vi "BMU参数读取-Auto.vi"(7 "Socket":dbl, 8 "CAN端口":u16(ring), 9 "设备索引号":u16(ring), 10 "CAN卡类型":u32(ring)=21, 11 "从板号":u8=1) -> (3 "成功?":bool)   [LabVIEW 2013] (continued)
                                n1965 = control-ref of="二维码信息"() -> (w3309:refnum<vi>)
                                n1966 = local write "主板数据"(w3310) -> ()
                                }
                                frame #1 {
                                n1967 = control-ref of="主板数据"() -> (w3321:refnum<vi>)
                                }
                                }
                                }
                                frame "从板" {
                                n1968 = stacked-sequence {
                                tunnel: [_ w3333] -> w3322
                                frame #0 {
                                n1969 = control-ref of="从板号"() -> (w3327:refnum<vi>)
                                n1970 = control-ref of="项目信息 2"() -> (w3328:refnum<vi>)
                                n1971 = control-ref of="电池组信息"() -> (w3326:refnum<vi>)
                                n1972 = control-ref of="加热控制参数"() -> (w3329:refnum<vi>)
                                n1973 = control-ref of="一级故障(从板)"() -> (w3330:refnum<vi>)
                                n1974 = control-ref of="二级故障(从板)"() -> (w3331:refnum<vi>)
                                n1975 = control-ref of="三级故障(从板)"() -> (w3332:refnum<vi>)
                                n1976 = control-ref of="均衡参数"() -> (w3325:refnum<vi>)
                                n1977 = local read "从板信息"() -> (w3324:T2)
                                n1978 = Bundle(cluster=w3324, "从板号"=w3327, "项目信息 2"=w3328, "加热控制参数"=w3329, "一级故障(从板)"=w3330, "二级故障(从板)"=w3331, "三级故障(从板)"=w3332, "电池组信息(从板)"=w3326, "均衡参数"=w3325) -> (w3323:T2)
                                n1979 = local write "从板信息"(w3323) -> ()
                                }
                                frame #1 {
                                n1980 = control-ref of="从板信息"() -> (w3333:refnum<vi>)
                                }
                                }
                                }
                              }
                              n1981 = control-ref of="BMU读取结果"() -> (w3294:refnum<vi>)
                              n1982 = control-ref of="二维码信息 2"() -> (w3296:refnum<vi>)
                              n1983 = control-ref of="结果"() -> (w3303:refnum<vi>)
                              n1984 = control-ref of="从板个数"() -> (w3299:refnum<vi>)
                              n1985 = call "输出数据解析.vi"("主板引用"=w3301, "错误代码"=w3306, "BMU读取结果"=w3294, "命令序号"=w3305, "输入数组"=w3304, "命令"=w3302, "从板引用"=w3300, "进度引用"=w3303, "板选择"=w3298, "从板个数"=w3299, "二维码信息"=w3297, "从板二维码信息"=w3296) -> ("写入超时"=→"写入超时":bool)  [unwired: 4 in, 3 out]
                            }
                            frame True {
                              n1986 = Index Array(array=w3334, index #1=0 ("索引"), index #2=1 ("索引")) -> (element #1=w3337:u8, element #2=w3338:u8)
                              n1987 = Join Numbers(hi=w3337, lo=w3338) -> ((hi.lo)=w3336:u16)
                              n1988 = Number To Hexadecimal String(2:w3336) -> (0:w3335:string)  [unwired: 1 out]
                              n1989 = control-ref of="结果"() -> (w3343:refnum<vi>)
                              n1990 = Concatenate Strings("0x" ("字符串"), w3335) -> (w3344:string)
                              n1991 = Build Array(w3344) -> (w3345:string[])
                              n1992 = call "表格编辑.vi"("新元素/子数组"=w3345, "活动单元格:单元格背景色"=u32 16740749, "MCListbox引用句柄"=w3343) -> ()  [unwired: 9 out]
                            }
                          }
                          n1993 = global write "EV05全局变量1.vi" "流控帧 2"(FALSE ("流控帧 2")) -> ()
                          n1994 = global write "EV05全局变量1.vi" "输出数组"(i32[] []) -> ()
                          n1995 = local write "控制1"(FALSE ("控制1")) -> ()
                          n1996 = local write "消除"(FALSE ("消除")) -> ()
                        }
                      }
                    }
                    frame True {
                      # "写参数判定"
                      n1997 = And(x="控制1", y=w3351) -> (x .and. y?=w3348:bool)
                      n1998 = case shown="真" w3348 {
                        tunnel: w3350 -> [_ w3358]
                        tunnel: w3349 -> [_ w3355]
                        frame False {
                        }
                        frame True {
                          n1999 = call <vilib>:"Unset Busy.vi"() -> ()  [unwired: 2 in, 10 out]
                          n2000 = case shown="\"主板\", 默认" w3355 {
                            tunnel: [w3359 w3360] -> w3357
                            frame "主板", Default {
                              n2001 = local read "主板选项"() -> (w3359:string)
                            }
                            frame "从板" {
                              n2002 = local read "从板选项"() -> (w3360:string)
                            }
                          }
                          n2003 = control-ref of="结果"() -> (w3356:refnum<vi>)
                          n2004 = call "输入数据判定.vi"("主从选择"=w3355, "主板选项"=w3357, "进度引用"=w3356, "错误代码"=w3358) -> ()  [unwired: 3 in, 5 out]
                          n2005 = global write "EV05全局变量1.vi" "流控帧 2"(FALSE ("流控帧 2")) -> ()
                          n2006 = local write "控制1"(FALSE ("控制1")) -> ()
                          n2007 = local write "消除"(FALSE ("消除")) -> ()
                        }
                      }
                      n2008 = global write "EV05全局变量1.vi" "输出数组"(i32[] []) -> ()
                    }
                  }
                }
                frame "版本读取" {
                  n2009 = local read "命令序号"() -> (w3361:u8)
                  n2010 = local read "从板板号"() -> (w3364:u8)
                  n2011 = local read "控制1"() -> (w3365:bool)
                  n2012 = call "多帧接收机制(EV05).vi"("can卡类型"=w3372, "设备索引号"=w3371, "CAN端口"=w3370, "VCI_Receive"=w3369, "命令"=w3368, "板号"=w3364, "命令序号"=w3361) -> ("错误信号"=w3362:bool, "输出数组"=w3373:u8[], "读错误代码"=w3363:u8[], "结束信号"=w3367:bool)  [unwired: 3 in, 6 out]
                  n2013 = And(x=w3365, y=w3367) -> (x .and. y?=w3366:bool)
                  n2014 = case shown="真" w3366 {
                    tunnel: w3373 -> [_ w3381]
                    tunnel: w3361 -> [_ w3380]
                    tunnel: w3368 -> [_ w3379]
                    tunnel: w3363 -> [_ w3375]
                    tunnel: w3362 -> [_ w3374]
                    frame False {
                    }
                    frame True {
                      n2015 = case shown="假" w3374 {
                        tunnel: w3381 -> [w3385 _]
                        tunnel: w3380 -> [w3384 _]
                        tunnel: w3379 -> [w3383 _]
                        tunnel: w3375 -> [w3382 w3609]
                        frame False {
                          n2016 = case shown="89" w3383 {
                            tunnel: w3384 -> [_ w3388]
                            tunnel: w3385 -> [_ w3387]
                            tunnel: w3382 -> [_ _]
                            frame 0, Default {
                            }
                            frame 137 {
                              n2017 = case shown="1" w3388 {
                                tunnel: w3387 -> [_ w3416 w3460 w3480 w3607]
                                frame 0, Default {
                                }
                                frame 1 {
                                w3398 = "." ("字符串")
                                n2018 = Array Subset(array=w3416, index=0 ("索引"), length=14 ("长度")) -> (w3429:u8[])
                                n2019 = Index Array(array=w3416, index=14 ("索引")) -> (element=w3419:u8)
                                n2020 = Index Array(array=w3416, index #1=15 ("索引"), index #2=16 ("索引")) -> (element #1=w3425:u8, element #2=w3426:u8)
                                n2021 = Index Array(array=w3416, index #1=17 ("索引"), index #2=18 ("索引")) -> (element #1=w3420:u8, element #2=w3421:u8)
                                n2022 = call "数组去零.vi"("输入"=w3429) -> ("输出"=w3404:dbl[])
                                n2023 = Join Numbers(hi=w3420, lo=w3421) -> ((hi.lo)=w3417:u16)
                                n2024 = Join Numbers(hi=w3425, lo=w3426) -> ((hi.lo)=w3418:u16)
                                n2025 = Number To Decimal String(number=w3419) -> (decimal integer string=w3411:string)  [unwired: 1 out]
                                n2026 = Byte Array To String(unsigned byte array=w3404) -> (string=w3403:string)
                                n2027 = Number To Decimal String(number=w3417) -> (decimal integer string=w3399:string)  [unwired: 1 out]
                                n2028 = Number To Decimal String(number=w3418) -> (decimal integer string=w3410:string)  [unwired: 1 out]
                                n2029 = Array Subset(array=w3416, index=21 ("索引"), length=7 ("长度")) -> (w3413:u8[])
                                n2030 = Concatenate Strings("V" ("字符串"), w3411, w3398, w3410, w3398, w3399) -> (w3408:string)
                                n2031 = call "数组去零.vi"("输入"=w3413) -> ("输出"=w3396:dbl[])
                                n2032 = Byte Array To String(unsigned byte array=w3396) -> (string=w3394:string)
                                n2033 = call <vilib>:"Space Constant.vi"() -> ("String"=w3395:string)
                                n2034 = Equal?(x=w3394, y=w3395) -> (x = y?=w3400:bool)
                                n2035 = Concatenate Strings("-" ("字符串"), w3394) -> (w3401:string)
                                n2036 = Select(t=w3395, s=w3400, f=w3401) -> (s? t:f=w3397:string)
                                n2037 = Concatenate Strings(w3403, "-" ("字符串"), w3408, w3397) -> (w3390:string)
                                n2038 = local read "项目软件版本"() -> (w3392:string[])
                                n2039 = local read "从板板号"() -> (w3389:u8)
                                n2040 = local write "项目软件版本号"(w3390) -> ()
                                n2041 = Replace Array Subset(array=w3392, new element=w3390, index=w3389) -> (w3391:string[])
                                n2042 = control-ref of="结果"() -> (w3407:refnum<vi>)
                                n2043 = local write "项目软件版本"(w3391) -> ()
                                n2044 = Build Array("项目软件版本     读取完成" ("读取结果")) -> (w3405:string[])
                                n2045 = call "表格编辑(版本读取).vi"("新元素/子数组"=w3405, "活动单元格:单元格背景色"=u32 6618880, "MCListbox引用句柄"=w3407) -> ()  [unwired: 9 out]
                                }
                                frame 2 {
                                w3443 = ""
                                w3440 = "." ("字符串")
                                n2046 = Array Subset(array=w3460, index=0 ("索引"), length=14 ("长度")) -> (w3448:u8[])
                                n2047 = Index Array(array=w3460, index=14 ("索引")) -> (element=w3463:u8)
                                n2048 = Index Array(array=w3460, index #1=15 ("索引"), index #2=16 ("索引")) -> (element #1=w3469:u8, element #2=w3470:u8)
                                n2049 = Index Array(array=w3460, index #1=17 ("索引"), index #2=18 ("索引")) -> (element #1=w3464:u8, element #2=w3465:u8)
                                n2050 = Join Numbers(hi=w3464, lo=w3465) -> ((hi.lo)=w3461:u16)
                                n2051 = Join Numbers(hi=w3469, lo=w3470) -> ((hi.lo)=w3462:u16)
                                n2052 = Number To Decimal String(number=w3461) -> (decimal integer string=w3441:string)  [unwired: 1 out]
                                n2053 = call "数组去零.vi"("输入"=w3448) -> ("输出"=w3447:dbl[])
                                n2054 = Number To Decimal String(number=w3463) -> (decimal integer string=w3455:string)  [unwired: 1 out]
                                n2055 = Number To Decimal String(number=w3462) -> (decimal integer string=w3454:string)  [unwired: 1 out]
                                n2056 = Array Subset(array=w3460, index=21 ("索引"), length=7 ("长度")) -> (w3457:u8[])
                                n2057 = Byte Array To String(unsigned byte array=w3447) -> (string=w3442:string)
                                n2058 = call "数组去零.vi"("输入"=w3457) -> ("输出"=w3439:dbl[])
                                n2059 = Concatenate Strings("V" ("字符串"), w3455, w3440, w3454, w3440, w3441) -> (w3452:string)
                                n2060 = Byte Array To String(unsigned byte array=w3439) -> (string=w3437:string)
                                n2061 = Equal?(x=w3443, y=w3437) -> (x = y?=w3444:bool)
                                n2062 = Concatenate Strings("-" ("字符串"), w3437) -> (w3445:string)
                                n2063 = Select(t=w3443, s=w3444, f=w3445) -> (s? t:f=w3438:string)
                                n2064 = Concatenate Strings(w3442, "-" ("字符串"), w3452, w3438) -> (w3433:string)
                                n2065 = local read "平台软件版本"() -> (w3435:string[])
                                n2066 = local read "从板板号"() -> (w3432:u8)
                                n2067 = local write "平台软件版本号"(w3433) -> ()
                                n2068 = Replace Array Subset(array=w3435, new element=w3433, index=w3432) -> (w3434:string[])
                                n2069 = control-ref of="结果"() -> (w3450:refnum<vi>)
                                n2070 = local write "平台软件版本"(w3434) -> ()
                                n2071 = Build Array("平台软件版本     读取完成" ("读取结果")) -> (w3449:string[])
                                n2072 = call "表格编辑(版本读取).vi"("新元素/子数组"=w3449, "活动单元格:单元格背景色"=u32 6618880, "MCListbox引用句柄"=w3450) -> ()  [unwired: 1 in, 8 out]
                                }
                                frame 3 {
                                n2073 = Index Array(array=w3480, index #1=0 ("索引"), index #2=1 ("索引")) -> (element #1=w3476:u8, element #2=w3477:u8)
                                n2074 = Join Numbers(hi=w3476, lo=w3477) -> ((hi.lo)=w3475:u16)
                                n2075 = case shown="99, 默认" w3475 {
                                tunnel: w3480 -> [w3483 _ w3517]
                                tunnel: w3475 -> [_ _ w3495]
                                frame 0 {
                                n2076 = Index Array(array=w3483, index #1=2 ("索引"), index #2=3 ("索引")) -> (element #1=w3487:u8, element #2=w3486:u8)
                                n2077 = Join Numbers(hi=w3487, lo=w3486) -> ((hi.lo)=w3482:u16)
                                n2078 = for {
                                N: w3482 -> [_]
                                tunnel: w3483 -> [w3492]
                                tunnel: [w3488] -> w3481 mode=indexing
                                i -> [w3491]
                                n2079 = Add(x=w3491, y=4) -> (x+y=w3489:i32)
                                n2080 = Index Array(array=w3492, index=w3489) -> (element=w3488:u8)
                                }
                                "MODEL号" <- w3481
                                }
                                frame 99, Default {
                                }
                                frame 1..40 {
                                w3500 = ""
                                w3521 = "." ("字符串")
                                n2081 = Array Subset(array=w3517, index=2 ("索引"), length=14 ("长度")) -> (w3506:u8[])
                                n2082 = Index Array(array=w3517, index=16 ("索引")) -> (element=w3529:u8)
                                n2083 = Index Array(array=w3517, index #1=17 ("索引"), index #2=18 ("索引")) -> (element #1=w3535:u8, element #2=w3536:u8)
                                n2084 = Index Array(array=w3517, index #1=19 ("索引"), index #2=20 ("索引")) -> (element #1=w3530:u8, element #2=w3531:u8)
                                n2085 = Join Numbers(hi=w3530, lo=w3531) -> ((hi.lo)=w3527:u16)
                                n2086 = Join Numbers(hi=w3535, lo=w3536) -> ((hi.lo)=w3528:u16)
                                n2087 = Number To Decimal String(number=w3495) -> (decimal integer string=w3515:string)  [unwired: 1 out]
                                n2088 = Number To Decimal String(number=w3529) -> (decimal integer string=w3523:string)  [unwired: 1 out]
                                n2089 = call "数组去零.vi"("输入"=w3506) -> ("输出"=w3505:dbl[])
                                n2090 = Number To Decimal String(number=w3528) -> (decimal integer string=w3522:string)  [unwired: 1 out]
                                n2091 = Number To Decimal String(number=w3527) -> (decimal integer string=w3520:string)  [unwired: 1 out]
                                n2092 = Byte Array To String(unsigned byte array=w3505) -> (string=w3507:string)
                                n2093 = Concatenate Strings("第" ("读取结果"), w3515, "模块" ("字符串"), "     读取完成" ("读取结果")) -> (w3508:string)
                                n2094 = Concatenate Strings("V" ("字符串"), w3523, w3521, w3522, w3521, w3520) -> (w3518:string)
                                n2095 = control-ref of="结果"() -> (w3511:refnum<vi>)
                                n2096 = Array Subset(array=w3517, index=23 ("索引"), length=7 ("长度")) -> (w3504:u8[])
                                n2097 = call "数组去零.vi"("输入"=w3504) -> ("输出"=w3499:dbl[])
                                n2098 = Byte Array To String(unsigned byte array=w3499) -> (string=w3496:string)
                                n2099 = Build Array(w3508) -> (w3510:string[])
                                n2100 = control-ref of="模块软件版本 2"() -> (w3512:refnum<vi>)
                                n2101 = local read "模块软件版本"() -> (w3513:T1)
                                n2102 = Equal?(x=w3500, y=w3496) -> (x = y?=w3501:bool)
                                n2103 = call "表格编辑(版本读取).vi"("新元素/子数组"=w3510, "活动单元格:单元格背景色"=u32 6618880, "MCListbox引用句柄"=w3511) -> ()  [unwired: 1 in, 8 out]
                                n2104 = Concatenate Strings("-" ("字符串"), w3496) -> (w3502:string)
                                n2105 = Select(t=w3500, s=w3501, f=w3502) -> (s? t:f=w3498:string)
                                n2106 = Concatenate Strings(w3507, "-" ("字符串"), w3518, w3498) -> (w3497:string)
                                n2107 = case shown="30" w3495 {
                                tunnel: [_ "VERSIONM" "BCUMCAL" "BMUMCAL" "BMURMCAL" "BCUCMCAL" "BCUDMCAL" "SCH" "BSW" "CDD" "DATALAYER" "DATAANALYSIS" "SOC" "SOH" "SOF" "INTRES" "INTCAN" "CARCAN" "CHGCANL" "THM" "CHGM" "HVM" "LVM" "BALM" "SAFEM" "RUNMODEM" "RELAY" "DO" "GBCHGDET" "SUPPLYPOWGDET" "SUMVDET" "CURDET" "TEMPERDET" "CELLVDET" "ISODET" "AI" "DI" "SYSCONF" "ECUCONF"] -> w3494
                                frame 0, Default {
                                }
                                frame 1 {
                                }
                                frame 2 {
                                }
                                frame 3 {
                                }
                                frame 4 {
                                }
                                frame 5 {
                                }
                                frame 6 {
                                }
                                frame 7 {
                                }
                                frame 8 {
                                }
                                frame 9 {
                                }
                                frame 10 {
                                }
                                frame 11 {
                                }
                                frame 12 {
                                }
                                frame 13 {
                                }
                                frame 14 {
                                }
                                frame 15 {
                                }
                                frame 16 {
                                }
                                frame 17 {
                                }
                                frame 18 {
                                }
                                frame 19 {
                                }
                                frame 20 {
                                }
                                frame 21 {
                                }
                                frame 22 {
                                }
                                frame 23 {
                                }
                                frame 24 {
                                }
                                frame 25 {
                                }
                                frame 26 {
                                }
                                frame 27 {
                                }
                                frame 28 {
                                }
                                frame 29 {
                                }
                                frame 30 {
                                }
                                frame 31 {
                                }
                                frame 32 {
                                }
                                frame 33 {
                                }
                                frame 34 {
                                }
                                frame 35 {
                                }
                                frame 36 {
                                }
                                frame 37 {
                                }
                                frame 38 {
                                }
                                }
                                n2108 = case shown="\"全部读取\"" w3513 {
                                tunnel: w3497 -> [w3580 w3588]
                                tunnel: w3495 -> [w3584 w3593]
                                tunnel: w3512 -> [w3586 w3594]
                                tunnel: w3494 -> [w3585 w3592]
                                frame "全部读取" {
                                n2109 = Number To Decimal String(number=w3584) -> (decimal integer string=w3583:string)  [unwired: 1 out]
                                n2110 = Concatenate Strings(w3583, "-" ("元素"), w3585) -> (w3581:string)
                                n2111 = Build Array(w3581, w3580) -> (w3579:string[])
                                n2112 = call "表格编辑(模块版本).vi"("新元素/子数组"=w3579, "MCListbox引用句柄"=w3586) -> ()  [unwired: 1 in, 9 out]
                                }
                                frame "BCUMCAL", Default {
                                n2113 = Number To Decimal String(number=w3593) -> (decimal integer string=w3591:string)  [unwired: 1 out]
                                n2114 = Concatenate Strings(w3591, "-" ("元素"), w3592) -> (w3589:string)
                                n2115 = Build Array(w3589, w3588) -> (w3587:string[])
                                n2116 = call "表格编辑(模块版本).vi"("新元素/子数组"=w3587, "MCListbox引用句柄"=w3594) -> ()  [unwired: 1 in, 9 out]
                                }
                                }
                                }
                                }
                                }
                                frame 4 {
                                n2117 = Array Subset(array=w3607, length=12 ("长度")) -> (w3605:u8[])  [unwired: 1 in]
                                n2118 = Byte Array To String(unsigned byte array=w3605) -> (string=w3604:string)
                                n2119 = call <vilib>:"Trim Whitespace.vi"("string"=w3604) -> ("trimmed string"=w3596:string)  [unwired: 1 in]
                                n2120 = local read "从板板号"() -> (w3595:u8)
                                n2121 = local write "硬件版本号"(w3596) -> ()
                                n2122 = local read "硬件版本"() -> (w3597:string[])
                                n2123 = Replace Array Subset(array=w3597, new element=w3596, index=w3595) -> (w3598:string[])
                                n2124 = local write "硬件版本"(w3598) -> ()
                                n2125 = global write "EV05全局变量1.vi" "写入超时"(TRUE ("写入超时")) -> ()
                                n2126 = control-ref of="结果"() -> (w3602:refnum<vi>)
                                n2127 = Build Array("硬件版本     读取完成" ("读取结果")) -> (w3601:string[])
                                n2128 = call "表格编辑(版本读取).vi"("新元素/子数组"=w3601, "活动单元格:单元格背景色"=u32 6618880, "MCListbox引用句柄"=w3602) -> ()  [unwired: 9 out]
                                }
                              }
                              n2129 = global write "EV05全局变量1.vi" "写入超时"(TRUE ("写入超时")) -> ()
                            }
                          }
                        }
                        frame True {
                          n2130 = Index Array(array=w3609, index #1=0 ("索引"), index #2=1 ("索引")) -> (element #1=w3614:u8, element #2=w3615:u8)
                          n2131 = Join Numbers(hi=w3614, lo=w3615) -> ((hi.lo)=w3613:u16)
                          n2132 = Number To Hexadecimal String(2:w3613) -> (0:w3612:string)  [unwired: 1 out]
                          n2133 = control-ref of="结果"() -> (w3611:refnum<vi>)
                          n2134 = Concatenate Strings("0x" ("字符串"), w3612) -> (w3619:string)
                          n2135 = Build Array(w3619) -> (w3610:string[])
                          n2136 = call "表格编辑(版本读取).vi"("新元素/子数组"=w3610, "活动单元格:单元格背景色"=u32 16740749, "MCListbox引用句柄"=w3611) -> ()  [unwired: 9 out]
                        }
                      }
                      n2137 = global write "EV05全局变量1.vi" "流控帧 2"(FALSE ("流控帧 2")) -> ()
                      n2138 = local write "控制1"(FALSE ("控制1")) -> ()
                      n2139 = local write "消除"(FALSE ("消除")) -> ()
                      n2140 = call <vilib>:"Unset Busy.vi"() -> ()  [unwired: 2 in, 10 out]
                    }
                  }
                }
                frame "其它诊断" {
                  n2141 = local read "命令序号"() -> (w3621:u8)
                  n2142 = call "多帧接收机制(EV05).vi"("can卡类型"=w3628, "设备索引号"=w3627, "CAN端口"=w3626, "VCI_Receive"=w3625, "命令"=w3623, "板号"=w3624, "命令序号"=w3621) -> ("错误代码"=w3630:i32, "输出数组"=w3622:u8[], "读错误代码"=w3620:u8[], "结束信号"=w3629:bool)  [unwired: 3 in, 6 out]
                  n2143 = case shown="真" w3629 {
                    tunnel: w3631 -> [_ w3632]
                    tunnel: w3630 -> [_ _]
                    tunnel: w3622 -> [_ w3633]
                    tunnel: w3621 -> [_ w3636]
                    tunnel: w3620 -> [_ w3634]
                    frame False {
                    }
                    frame True {
                      n2144 = Insert Into Array(array=w3634, new element=w3633) -> (w3635:u8[])  [unwired: 1 in]
                      n2145 = case shown="1" w3636 {
                        tunnel: w3635 -> [_ w3645 w3731]
                        tunnel: w3632 -> [_ _ w3726]
                        frame 0, Default {
                        }
                        frame 1 {
                          n2146 = Index Array(array=w3645) -> (element #1=w3644:u8, element #2=w3643:u8, element #3=w3642:u8)  [unwired: 3 in]
                          n2147 = Join Numbers(hi=w3643, lo=w3642) -> ((hi.lo)=w3641:u16)
                          n2148 = case shown="4" w3644 {
                            tunnel: w3645 -> [_ _ _ _ _ _ _ _ _ _]
                            tunnel: w3641 -> [_ w3648 w3656 w3666 w3676 w3686 w3696 w3706 w3716 _]
                            frame 0, Default {
                              n2149 = local write "继电器超时处理"(FALSE ("继电器超时处理")) -> ()
                            }
                            frame 1 {
                              n2150 = Equal To 0?(x=w3648) -> (x = 0?=w3647:bool)
                              n2151 = local write "正级继电器 12"(w3647) -> ()
                              n2152 = case shown="假" w3647 {
                                tunnel: w3648 -> [w3651 _]
                                frame False {
                                n2153 = local read "正级继电器"() -> (w3653:bool)
                                n2154 = Number To Hexadecimal String(2:w3651) -> (0:w3650:string)  [unwired: 1 out]
                                n2155 = local write "继电器超时处理"(TRUE ("继电器超时处理")) -> ()
                                n2156 = Not(x=w3653) -> (.not. x?=w3652:bool)
                                n2157 = Concatenate Strings("继电器操作失败,0x" ("消息"), w3650) -> ()  [unwired: 1 out]
                                n2158 = local write "正级继电器"(w3652) -> ()
                                }
                                frame True {
                                (unwired) "继电器操作成功!\n继电器操作成功!\n继电器操作成功!"
                                }
                              }
                            }
                            frame 2 {
                              n2159 = Equal To 0?(x=w3656) -> (x = 0?=w3655:bool)
                              n2160 = case shown="假" w3655 {
                                tunnel: w3656 -> [w3662 _]
                                tunnel: [w3660 "继电器操作成功!\n继电器操作成功!\n继电器操作成功!"] -> _
                                frame False {
                                n2161 = local read "负级继电器"() -> (w3658:bool)
                                n2162 = Number To Hexadecimal String(2:w3662) -> (0:w3661:string)  [unwired: 1 out]
                                n2163 = local write "继电器超时处理"(TRUE ("继电器超时处理")) -> ()
                                n2164 = Not(x=w3658) -> (.not. x?=w3659:bool)
                                n2165 = Concatenate Strings("继电器操作失败,0x" ("消息"), w3661) -> (w3660:string)
                                n2166 = local write "负级继电器"(w3659) -> ()
                                }
                                frame True {
                                }
                              }
                              n2167 = local write "正级继电器 2"(w3655) -> ()
                            }
                            frame 3 {
                              n2168 = Equal To 0?(x=w3666) -> (x = 0?=w3665:bool)
                              n2169 = case shown="假" w3665 {
                                tunnel: w3666 -> [w3672 _]
                                tunnel: [w3670 "继电器操作成功!\n继电器操作成功!\n继电器操作成功!"] -> _
                                frame False {
                                n2170 = local read "预充电继电器"() -> (w3668:bool)
                                n2171 = Number To Hexadecimal String(2:w3672) -> (0:w3671:string)  [unwired: 1 out]
                                n2172 = local write "继电器超时处理"(TRUE ("继电器超时处理")) -> ()
                                n2173 = Not(x=w3668) -> (.not. x?=w3669:bool)
                                n2174 = Concatenate Strings("继电器操作失败,0x" ("消息"), w3671) -> (w3670:string)
                                n2175 = local write "预充电继电器"(w3669) -> ()
                                }
                                frame True {
                                }
                              }
                              n2176 = local write "正级继电器 3"(w3665) -> ()
                            }
                            frame 4 {
                              n2177 = Equal To 0?(x=w3676) -> (x = 0?=w3675:bool)
                              n2178 = case shown="假" w3675 {
                                tunnel: w3676 -> [w3682 _]
                                tunnel: [w3680 "继电器操作成功!\n继电器操作成功!\n继电器操作成功!"] -> _
                                frame False {
                                n2179 = local read "加热继电器"() -> (w3679:bool)
                                n2180 = Number To Hexadecimal String(2:w3682) -> (0:w3681:string)  [unwired: 1 out]
                                n2181 = local write "继电器超时处理"(TRUE ("继电器超时处理")) -> ()
                                n2182 = Not(x=w3679) -> (.not. x?=w3678:bool)
                                n2183 = Concatenate Strings("继电器操作失败,0x" ("消息"), w3681) -> (w3680:string)
                                n2184 = local write "加热继电器"(w3678) -> ()
                                }
                                frame True {
                                }
                              }
                              n2185 = local write "正级继电器 5"(w3675) -> ()
                            }
                            frame 5 {
                              n2186 = Equal To 0?(x=w3686) -> (x = 0?=w3685:bool)
                              n2187 = case shown="假" w3685 {
                                tunnel: w3686 -> [w3692 _]
                                tunnel: [w3690 "继电器操作成功!\n继电器操作成功!\n继电器操作成功!"] -> _
                                frame False {
                                n2188 = local read "充电继电器"() -> (w3688:bool)
                                n2189 = Number To Hexadecimal String(2:w3692) -> (0:w3691:string)  [unwired: 1 out]
                                n2190 = local write "继电器超时处理"(TRUE ("继电器超时处理")) -> ()
                                n2191 = Not(x=w3688) -> (.not. x?=w3689:bool)
                                n2192 = Concatenate Strings("继电器操作失败,0x" ("消息"), w3691) -> (w3690:string)
                                n2193 = local write "充电继电器"(w3689) -> ()
                                }
                                frame True {
                                }
                              }
                              n2194 = local write "正级继电器 4"(w3685) -> ()
                            }
                            frame 6 {
                              n2195 = Equal To 0?(x=w3696) -> (x = 0?=w3695:bool)
                              n2196 = local write "正级继电器 6"(w3695) -> ()
                              n2197 = case shown="假" w3695 {
                                tunnel: w3696 -> [w3702 _]
                                tunnel: [w3700 "继电器操作成功!\n继电器操作成功!\n继电器操作成功!"] -> _
                                frame False {
                                n2198 = local read "风机继电器"() -> (w3698:bool)
                                n2199 = Number To Hexadecimal String(2:w3702) -> (0:w3701:string)  [unwired: 1 out]
                                n2200 = local write "继电器超时处理"(TRUE ("继电器超时处理")) -> ()
                                n2201 = Not(x=w3698) -> (.not. x?=w3699:bool)
                                n2202 = Concatenate Strings("继电器操作失败,0x" ("消息"), w3701) -> (w3700:string)
                                n2203 = local write "风机继电器"(w3699) -> ()
                                }
                                frame True {
                                }
                              }
                            }
                            frame 7 {
                              n2204 = Equal To 0?(x=w3706) -> (x = 0?=w3705:bool)
                              n2205 = case shown="假" w3705 {
                                tunnel: w3706 -> [w3711 _]
                                tunnel: [w3709 "继电器操作成功!\n继电器操作成功!\n继电器操作成功!"] -> _
                                frame False {
                                n2206 = local read "加热继电器(从)"() -> (w3707:bool)
                                n2207 = Number To Hexadecimal String(2:w3711) -> (0:w3710:string)  [unwired: 1 out]
                                n2208 = Not(x=w3707) -> (.not. x?=w3708:bool)
                                n2209 = Concatenate Strings("继电器操作失败,0x" ("消息"), w3710) -> (w3709:string)
                                n2210 = local write "加热继电器(从)"(w3708) -> ()
                                }
                                frame True {
                                n2211 = local write "继电器超时处理"(TRUE ("继电器超时处理")) -> ()
                                }
                              }
                              n2212 = local write "正级继电器 7"(w3705) -> ()
                            }
                            frame 8 {
                              n2213 = Equal To 0?(x=w3716) -> (x = 0?=w3715:bool)
                              n2214 = case shown="假" w3715 {
                                tunnel: w3716 -> [w3721 _]
                                tunnel: [w3719 "继电器操作成功!\n继电器操作成功!\n继电器操作成功!"] -> _
                                frame False {
                                n2215 = local read "风机继电器(从)"() -> (w3717:bool)
                                n2216 = Number To Hexadecimal String(2:w3721) -> (0:w3720:string)  [unwired: 1 out]
                                n2217 = Not(x=w3717) -> (.not. x?=w3718:bool)
                                n2218 = Concatenate Strings("继电器操作失败,0x" ("消息"), w3720) -> (w3719:string)
                                n2219 = local write "风机继电器(从)"(w3718) -> ()
                                }
                                frame True {
                                n2220 = local write "继电器超时处理"(TRUE ("继电器超时处理")) -> ()
                                }
                              }
                              n2221 = local write "正级继电器 8"(w3715) -> ()
                            }
                            frame 85, 170 {
                              n2222 = local write "继电器超时处理"(TRUE ("继电器超时处理")) -> ()
                            }
                          }
                        }
                        frame 2 {
                          n2223 = Index Array(array=w3731) -> (element #1=w3730:u8, element #2=w3729:u8, element #3=w3728:u8)  [unwired: 3 in]
                          n2224 = Join Numbers(hi=w3729, lo=w3728) -> ((hi.lo)=w3727:u16)
                          n2225 = case shown="2" w3730 {
                            tunnel: w3731 -> [_ _ _]
                            tunnel: w3727 -> [_ w3735 w3749]
                            tunnel: w3726 -> [_ w3734 _]
                            frame 0, Default {
                              n2226 = local write "继电器超时处理"(FALSE ("继电器超时处理")) -> ()
                            }
                            frame 1 {
                              n2227 = Equal To 0?(x=w3735) -> (x = 0?=w3733:bool)
                              n2228 = case shown="假" w3733 {
                                tunnel: w3735 -> [w3741 _]
                                tunnel: [w3739 "DO控制操作成功!\nDO控制操作成功!\nDO控制操作成功!"] -> _
                                tunnel: w3734 -> [w3738 _]
                                frame False {
                                n2229 = case shown="\"主板\", 默认" w3738 {
                                frame "主板", Default {
                                n2230 = local read "DO1"() -> (w3744:bool)
                                n2231 = Not(x=w3744) -> (.not. x?=w3743:bool)
                                n2232 = local write "DO1"(w3743) -> ()
                                }
                                frame "从板" {
                                n2233 = local read "DO1 2"() -> (w3746:bool)
                                n2234 = Not(x=w3746) -> (.not. x?=w3745:bool)
                                n2235 = local write "DO1 2"(w3745) -> ()
                                }
                                }
                                n2236 = Number To Hexadecimal String(2:w3741) -> (0:w3740:string)  [unwired: 1 out]
                                n2237 = Concatenate Strings("DO控制操作失败,0x" ("消息"), w3740) -> (w3739:string)
                                }
                                frame True {
                                }
                              }
                              n2238 = case shown="\"从板\"" w3734 {
                                tunnel: w3733 -> [w3736 w3737]
                                frame "主板", Default {
                                n2239 = local write "正级继电器 9"(w3736) -> ()
                                }
                                frame "从板" {
                                n2240 = local write "正级继电器 11"(w3737) -> ()
                                }
                              }
                            }
                            frame 2 {
                              n2241 = Equal To 0?(x=w3749) -> (x = 0?=w3748:bool)
                              n2242 = case shown="假" w3748 {
                                tunnel: w3749 -> [w3754 _]
                                tunnel: [w3752 "DO控制操作成功!\nDO控制操作成功!\nDO控制操作成功!"] -> _
                                frame False {
                                n2243 = Number To Hexadecimal String(2:w3754) -> (0:w3753:string)  [unwired: 1 out]
                                n2244 = local read "DO2"() -> (w3751:bool)
                                n2245 = Not(x=w3751) -> (.not. x?=w3750:bool)
                                n2246 = Concatenate Strings("DO控制操作失败,0x" ("消息"), w3753) -> (w3752:string)
                                n2247 = local write "DO2"(w3750) -> ()
                                }
                                frame True {
                                }
                              }
                              n2248 = local write "正级继电器 10"(w3748) -> ()
                            }
                          }
                        }
                      }
                      n2249 = local write "消除"(FALSE ("消除")) -> ()
                      n2250 = global write "EV05全局变量1.vi" "流控帧 2"(FALSE ("流控帧 2")) -> ()
                      n2251 = local write "控制1"(FALSE ("控制1")) -> ()
                      "继电器超时处理" <- TRUE ("控制1")
                    }
                  }
                }
                frame "高压板校正" {
                  n2252 = local read "命令序号"() -> (w3761:u8)
                  n2253 = call "多帧接收机制(EV05).vi"("can卡类型"=w3768, "设备索引号"=w3767, "CAN端口"=w3766, "VCI_Receive"=w3765, "命令"=w3763, "板号"=w3764, "命令序号"=w3761) -> ("错误信号"=w3757:bool, "错误代码"=w3770:i32, "输出数组"=w3762:u8[], "读错误代码"=w3760:u8[], "结束信号"=w3769:bool)  [unwired: 3 in, 5 out]
                  n2254 = local read "控制1"() -> (w3758:bool)
                  n2255 = And(x=w3758, y=w3769) -> (x .and. y?=w3759:bool)
                  n2256 = case shown="真" w3759 {
                    tunnel: w3771 -> [_ w3775]
                    tunnel: w3770 -> [_ _]
                    tunnel: w3762 -> [_ w3773]
                    tunnel: w3761 -> [_ w3774]
                    tunnel: w3760 -> [_ w3776]
                    tunnel: w3757 -> [_ w3777]
                    frame False {
                    }
                    frame True {
                      n2257 = case shown="假" w3777 {
                        tunnel: w3776 -> [_ w3987]
                        tunnel: w3775 -> [_ _]
                        tunnel: w3774 -> [w3782 _]
                        tunnel: w3773 -> [w3781 _]
                        frame False {
                          n2258 = case shown="2" w3782 {
                            tunnel: w3781 -> [_ w3787 w3821 w3851 w3878 w3905 w3932 w3959]
                            frame 0, Default {
                            }
                            frame 1 {
                              n2259 = for {
                                N: 10 -> [_]
                                tunnel: w3787 -> [w3804]
                                shift-right: [w3791] -> w3785
                                shift-left: string[] [] -> [w3793]
                                i -> [w3790]
                                w3798 = 8 ("索引")
                                w3802 = 2 ("y")
                                n2260 = Multiply(x=w3790, y=w3802) -> (x*y=w3803:i32)
                                n2261 = Array Subset(array=w3804, index=w3803, length=w3802) -> (w3801:u8[])
                                n2262 = Index Array(array=w3801) -> (element #1=w3800:u8, element #2=w3799:u8)  [unwired: 2 in]
                                n2263 = call "二进制解析-8.6.vi"("索引"=w3798, "数值"=w3800) -> ("低位子数组"=w3797:i32[])  [unwired: 1 in, 2 out]
                                n2264 = call "二进制解析-8.6.vi"("索引"=w3798, "数值"=w3799) -> ("低位子数组"=w3796:i32[])  [unwired: 1 in, 2 out]
                                n2265 = Insert Into Array(array=w3797, new element=w3796) -> (w3795:i32[])  [unwired: 1 in]
                                n2266 = case shown="2" w3790 {
                                tunnel: [6 15 9 4 2 0 2] -> w3789
                                frame 0, Default {
                                }
                                frame 1 {
                                }
                                frame 2 {
                                }
                                frame 3..5 {
                                }
                                frame 8, 9 {
                                }
                                frame 7 {
                                }
                                frame 6 {
                                }
                                }
                                n2267 = Reverse 1D Array(array=w3795) -> (reversed array=w3794:i32[])
                                n2268 = for {
                                N: w3789 -> [_]
                                tunnel: w3794 -> [w3816] mode=indexing
                                tunnel: [w3812] -> w3792 mode=indexing
                                n2269 = Equal To 0?(x=w3816) -> (x = 0?=w3815:bool)
                                n2270 = Select(t="无", s=w3815, f="故障") -> (s? t:f=w3812:string)
                                }
                                n2271 = Insert Into Array(array=w3793, new element=w3792) -> (w3791:string[])  [unwired: 1 in]
                              }
                              n2272 = call "详细故障分解.vi"("名称"=string[] ["上电自检异常(CellV)", "通讯异常(CellV)", "不更新(CellV)", "未校准(CellV)", "保留", "采样线路断路(CellV)", "18b20上电自检异常(T) ", "18b20通讯异常(T)", "18b20传感器丢失(T)", "18b20传感器无号(T)", "18b20温度异常跳变(T)", "18b20信号线对电源短路(T)", "18b20信号线对地短路(T)", "18b20 CRC校验异常(T)", "NTC上电自检异常(T)", "NTC通讯异常(T)", "NTC传感器丢失(T)", "NTC温度异常跳变(T)", "NTC信号线断路(T)", "NTC信号线对电源短(T)", "NTC信号线对地短路(T)", "上电自检异常(Curr)", "参数异常(Curr)", "不更新(Curr)", "未校准(Curr)", "采样线断开(Curr)", "电流零漂异常(Curr)", "传感器反接(Curr)", "读取实时电流故障(Curr)", "平均电流故障(Curr)", "自检异常(iso)", "前端检测电阻损坏(iso)", "不更新(iso)", "未校准(iso)", "上电自检异常(Sumv_in)", "通讯异常(Sumv_in)", "不更新(Sumv_in)", "未校准(Sumv_in)", "上电自检异常(Sumv_out)", "通讯异常(Sumv_out)", "不更新(Sumv_out)", "未校准(Sumv_out)", "系统时钟自检异常(Clock)", "系统时钟未校准(Clock)", "充电均衡模块不能开启", "充电均衡模块不能关闭", "放电均衡模块不能开启", "放电均衡模块不能关闭"], "故障输入口"=w3785) -> ("输出数组"=w3783:string[][])  [unwired: 1 in, 2 out]
                              n2273 = local write "电池故障"(w3783) -> ()
                            }
                            frame 2 {
                              n2274 = for {
                                N: 5 -> [_]
                                tunnel: w3821 -> [w3838]
                                shift-right: [w3825] -> w3819
                                shift-left: string[] [] -> [w3827]
                                i -> [w3823]
                                w3832 = 8 ("索引")
                                w3836 = 2 ("y")
                                n2275 = Multiply(x=w3823, y=w3836) -> (x*y=w3837:i32)
                                n2276 = Array Subset(array=w3838, index=w3837, length=w3836) -> (w3835:u8[])
                                n2277 = Index Array(array=w3835) -> (element #1=w3834:u8, element #2=w3833:u8)  [unwired: 2 in]
                                n2278 = call "二进制解析-8.6.vi"("索引"=w3832, "数值"=w3834) -> ("低位子数组"=w3831:i32[])  [unwired: 1 in, 2 out]
                                n2279 = call "二进制解析-8.6.vi"("索引"=w3832, "数值"=w3833) -> ("低位子数组"=w3830:i32[])  [unwired: 1 in, 2 out]
                                n2280 = Insert Into Array(array=w3831, new element=w3830) -> (w3829:i32[])  [unwired: 1 in]
                                n2281 = case shown="2" w3823 {
                                tunnel: [4 6 5] -> w3824
                                frame 0, Default {
                                }
                                frame 2 {
                                }
                                frame 4 {
                                }
                                }
                                n2282 = Reverse 1D Array(array=w3829) -> (reversed array=w3828:i32[])
                                n2283 = for {
                                N: w3824 -> [_]
                                tunnel: w3828 -> [w3846] mode=indexing
                                tunnel: [w3842] -> w3826 mode=indexing
                                n2284 = Equal To 0?(x=w3846) -> (x = 0?=w3845:bool)
                                n2285 = Select(t="无", s=w3845, f="故障") -> (s? t:f=w3842:string)
                                }
                                n2286 = Insert Into Array(array=w3827, new element=w3826) -> (w3825:string[])  [unwired: 1 in]
                              }
                              n2287 = call "详细故障分解.vi"("名称"=string[] ["自检异常(ee_cpu)", "存储空间满(ee_cpu)", "数据写入失败(ee_cpu)", "数据读取异常(ee_cpu)", "自检异常(ee_ext)", "存储空间满(ee_ext)", "数据写入失败(ee_ext)", "数据读取异常(ee_ext)", "自检异常(flash_ext)", "故障数据存储空间满(flash_ext)", "历史数据存储空间满(flash_ext)", "数据写入失败(flash_ext)", "数据读取失败(flash_ext)", "数据校验异常(flash_ext)", "自检异常(flash_cpu)", "存储空间满(flash_cpu)", "数据写入失败(flash_cpu)", "数据读取异常(flash_cpu)", "应用程序异常(cpu)", "应用程序下载异常(cpu)", "AD模块异常(cpu)", "RAM异常(cpu)", "CPU异常下电(cpu)"], "故障输入口"=w3819) -> ("输出数组"=w3817:string[][])  [unwired: 1 in, 2 out]
                              n2288 = local write "电池故障"(w3817) -> ()
                            }
                            frame 3 {
                              n2289 = for {
                                N: 5 -> [_]
                                tunnel: w3851 -> [w3868]
                                shift-right: [w3855] -> w3849
                                shift-left: string[] [] -> [w3857]
                                i -> [w3854]
                                w3862 = 8 ("索引")
                                w3866 = 2 ("y")
                                n2290 = Multiply(x=w3854, y=w3866) -> (x*y=w3867:i32)
                                n2291 = Array Subset(array=w3868, index=w3867, length=w3866) -> (w3865:u8[])
                                n2292 = Index Array(array=w3865) -> (element #1=w3864:u8, element #2=w3863:u8)  [unwired: 2 in]
                                n2293 = call "二进制解析-8.6.vi"("索引"=w3862, "数值"=w3864) -> ("低位子数组"=w3861:i32[])  [unwired: 1 in, 2 out]
                                n2294 = call "二进制解析-8.6.vi"("索引"=w3862, "数值"=w3863) -> ("低位子数组"=w3860:i32[])  [unwired: 1 in, 2 out]
                                n2295 = Insert Into Array(array=w3861, new element=w3860) -> (w3859:i32[])  [unwired: 1 in]
                                n2296 = Reverse 1D Array(array=w3859) -> (reversed array=w3858:i32[])
                                n2297 = for {
                                N: 6 -> [_]
                                tunnel: w3858 -> [w3873] mode=indexing
                                tunnel: [w3869] -> w3856 mode=indexing
                                n2298 = Equal To 0?(x=w3873) -> (x = 0?=w3872:bool)
                                n2299 = Select(t="无", s=w3872, f="故障") -> (s? t:f=w3869:string)
                                }
                                n2300 = Insert Into Array(array=w3857, new element=w3856) -> (w3855:string[])  [unwired: 1 in]
                              }
                              n2301 = call "详细故障分解.vi"("名称"=string[] ["初始化失败(CAN4)", "发送异常(CAN4)", "接收异常(CAN4)", "总线超时(CAN4)", "BUSOFF(CAN4)", "帧格式(CAN4)", "初始化异常(CAN0)", "发送异常(CAN0)", "接收异常(CAN0)", "总线超时(CAN0)", "BUSOFF(CAN0)", "帧格式(CAN0)", "初始化异常(CAN1)", "发送异常(CAN1)", "接收异常(CAN1)", "总线超时(CAN1)", "BUSOFF(CAN1)", "帧格式(CAN1)", "初始化失败(CAN2)", "发送异常(CAN2)", "接收异常(CAN2)", "总线超时(CAN2)", "BUSOFF(CAN2)", "帧格式(CAN2)", "初始化失败(CAN3)", "发送异常(CAN3)", "接收异常(CAN3)", "总线超时(CAN3)", "BUSOFF(CAN3)", "帧格式(CAN3)"], "故障输入口"=w3849) -> ("输出数组"=w3847:string[][])  [unwired: 1 in, 2 out]
                              n2302 = local write "电池故障"(w3847) -> ()
                            }
                            frame 4 {
                              n2303 = for {
                                N: 1 -> [_]
                                tunnel: w3878 -> [w3895]
                                shift-right: [w3882] -> w3876
                                shift-left: string[] [] -> [w3884]
                                i -> [w3881]
                                w3889 = 8 ("索引")
                                w3893 = 2 ("y")
                                n2304 = Multiply(x=w3881, y=w3893) -> (x*y=w3894:i32)
                                n2305 = Array Subset(array=w3895, index=w3894, length=w3893) -> (w3892:u8[])
                                n2306 = Index Array(array=w3892) -> (element #1=w3891:u8, element #2=w3890:u8)  [unwired: 2 in]
                                n2307 = call "二进制解析-8.6.vi"("索引"=w3889, "数值"=w3891) -> ("低位子数组"=w3888:i32[])  [unwired: 1 in, 2 out]
                                n2308 = call "二进制解析-8.6.vi"("索引"=w3889, "数值"=w3890) -> ("低位子数组"=w3887:i32[])  [unwired: 1 in, 2 out]
                                n2309 = Insert Into Array(array=w3888, new element=w3887) -> (w3886:i32[])  [unwired: 1 in]
                                n2310 = Reverse 1D Array(array=w3886) -> (reversed array=w3885:i32[])
                                n2311 = for {
                                N: 4 -> [_]
                                tunnel: w3885 -> [w3900] mode=indexing
                                tunnel: [w3896] -> w3883 mode=indexing
                                n2312 = Equal To 0?(x=w3900) -> (x = 0?=w3899:bool)
                                n2313 = Select(t="无", s=w3899, f="故障") -> (s? t:f=w3896:string)
                                }
                                n2314 = Insert Into Array(array=w3884, new element=w3883) -> (w3882:string[])  [unwired: 1 in]
                              }
                              n2315 = call "详细故障分解.vi"("名称"=string[] ["通讯协议版本不一致(soft)", "系统不同步(soft)", "软件版本不一致(soft)", "同硬件平台不兼容(soft)"], "故障输入口"=w3876) -> ("输出数组"=w3874:string[][])  [unwired: 1 in, 2 out]
                              n2316 = local write "电池故障"(w3874) -> ()
                            }
                            frame 5 {
                              n2317 = for {
                                N: 2 -> [_]
                                tunnel: w3905 -> [w3922]
                                shift-right: [w3909] -> w3903
                                shift-left: string[] [] -> [w3911]
                                i -> [w3908]
                                w3916 = 8 ("索引")
                                w3920 = 2 ("y")
                                n2318 = Multiply(x=w3908, y=w3920) -> (x*y=w3921:i32)
                                n2319 = Array Subset(array=w3922, index=w3921, length=w3920) -> (w3919:u8[])
                                n2320 = Index Array(array=w3919) -> (element #1=w3918:u8, element #2=w3917:u8)  [unwired: 2 in]
                                n2321 = call "二进制解析-8.6.vi"("索引"=w3916, "数值"=w3918) -> ("低位子数组"=w3915:i32[])  [unwired: 1 in, 2 out]
                                n2322 = call "二进制解析-8.6.vi"("索引"=w3916, "数值"=w3917) -> ("低位子数组"=w3914:i32[])  [unwired: 1 in, 2 out]
                                n2323 = Insert Into Array(array=w3915, new element=w3914) -> (w3913:i32[])  [unwired: 1 in]
                                n2324 = Reverse 1D Array(array=w3913) -> (reversed array=w3912:i32[])
                                n2325 = for {
                                N: 4 -> [_]
